vi "Diagnostics_Automation Example.vi"() -> ()   [LabVIEW 2015]
uses:
  Built/custom devices/Diagnostics Addon/Windows/Host Automation API/Diagnostics Host Automation API.lvlibp/Shared/Types/Command.ReadDTC.DTCs.ctl
  Built/custom devices/Diagnostics Addon/Windows/Host Automation API/Diagnostics Host Automation API.lvlibp
  Built/custom devices/Diagnostics Addon/Windows/Host Automation API/Diagnostics Host Automation API.lvlibp/Shared/Diagnostics Addon Shared.lvlib
panel:
  out "Active DTCs":T1[](array[typedef])
  out "error out":errorcluster
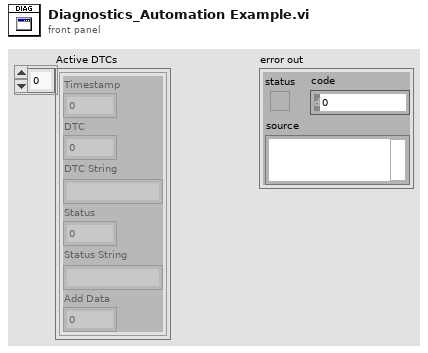
[diagram p1: front panel]
types:
  T1 = typedef "Diagnostics Host Automation API.lvlibp/Diagnostics Addon Shared.lvlib/Command.ReadDTC.DTCs.ctl" = cluster{"Timestamp":dbl, "DTC":dbl, "DTC String":string, "Status":dbl, "Status String":string, "Add Data":dbl}
  T2 = typedef "Diagnostics Host Automation API.lvlibp/Diagnostics Addon Shared.lvlib/HostAutomation.Ref.ctl" = cluster{"TCP Comm":T3, "DTCs":T5}
  T3 = typedef "Diagnostics Host Automation API.lvlibp/NI STM.lvlib/TCP Connection Info.ctl" = cluster{"connection ID":refnum<k5>, "meta data":T4[]}
  T4 = typedef "Diagnostics Host Automation API.lvlibp/NI STM.lvlib/MetaDataElement.ctl" = string
  T5 = typedef "Diagnostics Host Automation API.lvlibp/Diagnostics Addon Shared.lvlib/DTC.Codes.ctl" = cluster{"Value.Code":dbl[], "Value.String":string[], "Status.Code":dbl[], "Status.String":string[]}
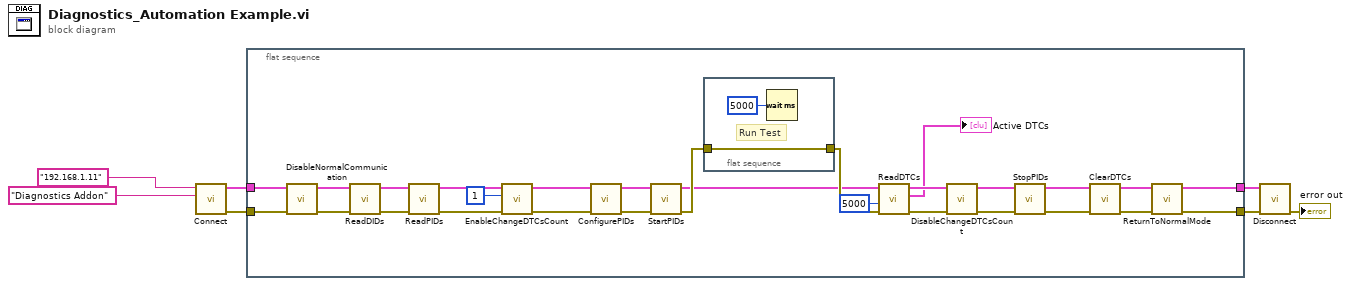
[diagram p0: block diagram]
diagram:
  n1 = call "Connect.vi"("Addon Name"="Diagnostics Addon" ("Address"), "Address"="192.168.1.11") -> ("error out"=w6:errorcluster, "Ref"=w3:T2)  [unwired: 8 in]
  n2 = flat-sequence {
    tunnel: [w26] -> w7
    tunnel: w6 -> [w30]
    tunnel: w3 -> [w18]
    tunnel: [w25] -> w1
    frame #0 {
      n3 = call "DisableNormalCommunication.vi"("error in (no error)"=w30, "Ref"=w18) -> ("error out"=w29:errorcluster, "Ref"=w17:T2)  [unwired: 8 in]
      n4 = call "ReadDIDs.vi"("error in (no error)"=w29, "Ref"=w17) -> ("error out"=w31:errorcluster, "Ref"=w16:T2)  [unwired: 8 in]
      n5 = call "ReadPIDs.vi"("error in (no error)"=w31, "Ref"=w16) -> ("error out"=w23:errorcluster, "Ref"=w15:T2)  [unwired: 8 in]
      n6 = call "EnableChangeDTCsCount.vi"("error in (no error)"=w23, "status mask"=u8 1, "Ref"=w15) -> ("error out"=w21:errorcluster, "Ref"=w14:T2)  [unwired: 7 in]
      n7 = call "ConfigurePIDs.vi"("error in (no error)"=w21, "Ref"=w14) -> ("error out"=w35:errorcluster, "Ref"=w13:T2)  [unwired: 8 in]
      n8 = call "StartPIDs.vi"("error in (no error)"=w35, "Ref"=w13) -> ("error out"=w33:errorcluster, "Ref"=w12:T2)  [unwired: 8 in]
      n9 = flat-sequence {
        tunnel: w33 -> [w36]
        tunnel: [w36] -> w32
        frame #0 {
          # "Run Test"
          n10 = Wait (ms)(milliseconds to wait=u32 5000) -> ()  [unwired: 1 out]
        }
      }
      n11 = call "ReadDTCs.vi"("error in (no error)"=w32, "timeout ms (1000)"=5000, "Ref"=w12) -> ("error out"=w20:errorcluster, "Active DTCs"=→"Active DTCs":T1[], "Ref"=w11:T2)  [unwired: 6 in]
      n12 = call "DisableChangeDTCsCount.vi"("error in (no error)"=w20, "Ref"=w11) -> ("error out"=w19:errorcluster, "Ref"=w10:T2)  [unwired: 8 in]
      n13 = call "StopPIDs.vi"("error in (no error)"=w19, "Ref"=w10) -> ("error out"=w24:errorcluster, "Ref"=w9:T2)  [unwired: 8 in]
      n14 = call "ClearDTCs.vi"("error in (no error)"=w24, "Ref"=w9) -> ("error out"=w28:errorcluster, "Ref"=w27:T2)  [unwired: 8 in]
      n15 = call "ReturnToNormalMode.vi"("error in (no error)"=w28, "Ref"=w27) -> ("error out"=w26:errorcluster, "Ref"=w25:T2)  [unwired: 8 in]
    }
  }
  n16 = call "Disconnect.vi"("error in"=w7, "Ref"=w1) -> ("error out"=→"error out":errorcluster)  [unwired: 9 in]
